vi "FT_GetComPortNumber.vi"(0 "Handle":u32) -> (5 "FT_Status":u32, 7 "Handle":u32, 8 "ComNumber":u32)   [LabVIEW 2010]
uses:
  FTD2XX.dll
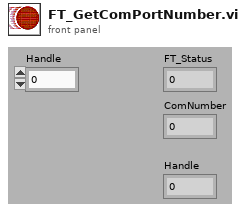
[diagram p1: front panel]
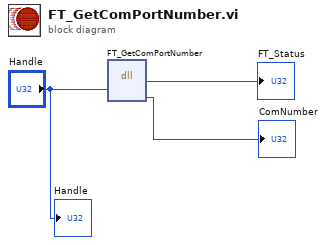
[diagram p0: block diagram]
diagram:
  n1 = dll-call lib="FTD2XX.dll" fn="FT_GetComPortNumber"("Handle"="Handle") -> ("FT_Status"=→"FT_Status":u32, "ComNumber"=→"ComNumber":i32)  [unwired: 5 in, 2 out]
  "Handle" <- "Handle"
